vi "CSV Reader.vi"(8 "error in":errorcluster, 11 "file (use dialog)":path) -> (0 "error out":errorcluster, 3 "Notes Array":dbl[](array[numeric]))   [LabVIEW 2018]
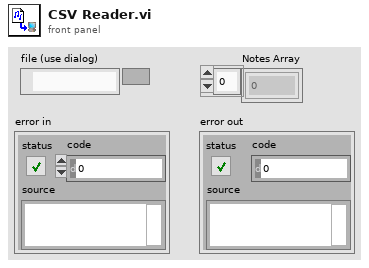
[diagram p1: front panel]
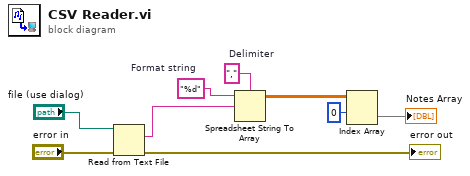
[diagram p0: block diagram]
diagram:
  w7 = "%d"  # Format string
  w3 = ","  # Delimiter
  n1 = Read from Text File(file (use dialog)="file (use dialog)", error in="error in") -> (text=w2:string, error out=→"error out":errorcluster)  [unwired: 2 in, 2 out]
  n2 = Spreadsheet String To Array(delimiter (Tab)=w3, format string=w7, spreadsheet string=w2) -> (array=w4:dbl[][])  [unwired: 1 in]
  n3 = Index Array "Index Array"(array=w4, index (row)=0) -> (element=→"Notes Array":dbl[])  [unwired: 1 in]
